vi "CreatePolynomial.vi"(6 "Save calibration":bool, 8 "Acquisition time (ms)":dbl=10000.0, 9 "Flyback (ms)":dbl=25.0, 10 "P(x)":dbl[](array[numeric])=[-0.257, 0.543, -0.0481, -0.0116] step=1e-10 format="%#.33f") -> (2 "Waveform Graph 2":dbl[](graph), 3 "Waveform Graph":dbl[](graph))   [LabVIEW 2020]
uses:
  <vilib>/Analysis/polynomials.llb/1D Polynomial Evaluation (DBL).vi
  <vilib>/Analysis/NI_AALPro.lvlib
panel:
  out "P(x) 2":dbl[](array[numeric])
  in  "Parameter string":string
  in  "Generate from string":bool
  out "size(s) 2":i32
  out "size(s)":i32
  out "x*y":dbl
  out "flyback min":dbl
  out "EndPosition":dbl
  out "InitialPosition":dbl
  # "=-0.257 + 0.543*F2 + -0.0481*F2^2 + -0.0116*F2^3"
  # "P(x) contains the real polynomial coefficients in ascending order of power."
  # "=-0.257 + 0.543*F2 + -0.0481*F2^2 + -0.0116*F2^3"
  # "D"
  # "C"
  # "B"
  # "A"
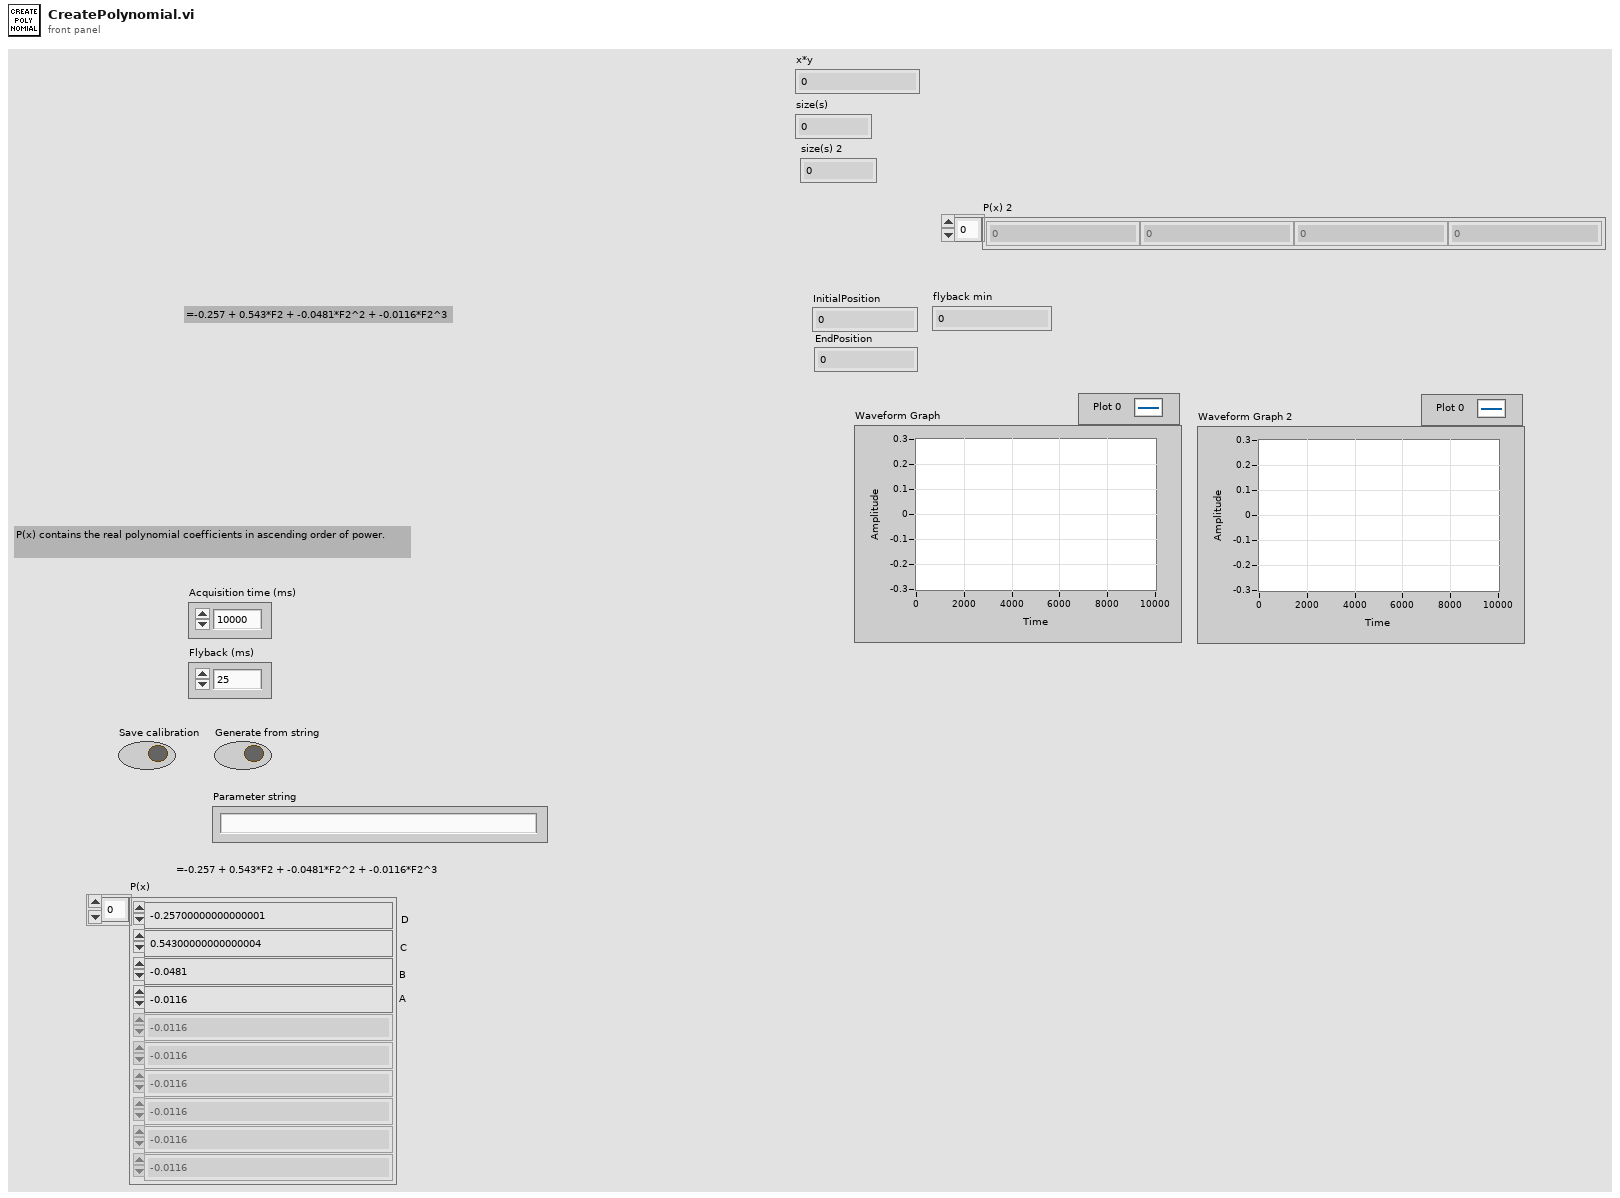
[diagram p1: front panel]
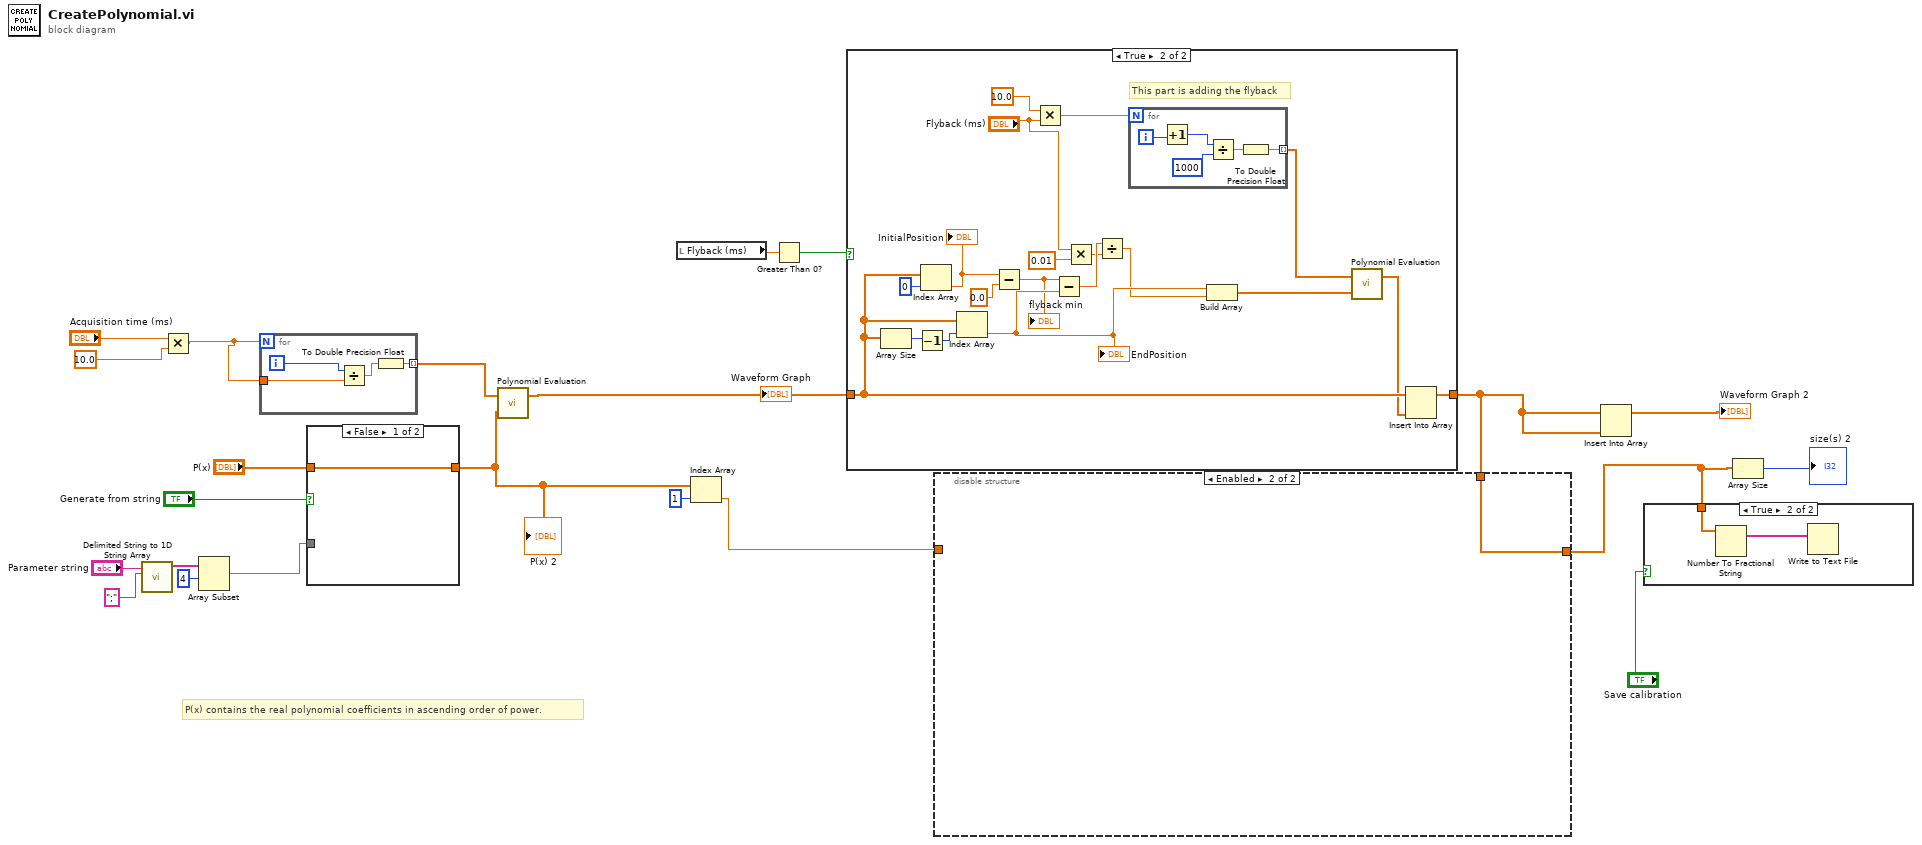
[diagram p0: block diagram]
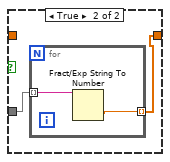
[diagram p3: hidden frame]
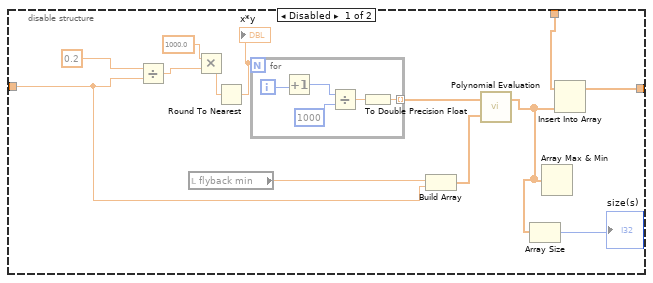
[diagram p4: hidden frame]
diagram:
  # "P(x) contains the real polynomial coefficients in ascending order of power."
  n1 = call <vilib>:"Delimited String to 1D String Array.vi"("delimiter"=";", "delimited string"="Parameter string") -> ("string array"=w6:string[])  [unwired: 9 in]
  n2 = Multiply(x="Acquisition time (ms)", y=10.0) -> (x*y=w18:dbl)
  n3 = Array Subset(array=w6, index=4) -> (w4:string[])  [unwired: 1 in]
  n4 = for {
    N: w18 -> [_]
    tunnel: [w26] -> w22 mode=indexing
    tunnel: w18 -> [w23]
    i -> [w25]
    n5 = Divide(x=w25, y=w23) -> (x/y=w24:dbl)
    n6 = To Double Precision Float(number=w24) -> (double precision float=w26:dbl)
  }
  n7 = case shown="False" "Generate from string" {
    tunnel: "P(x)" -> [w27 _]
    tunnel: [w27 w28] -> w9
    tunnel: w4 -> [_ w29]
    frame False {
    }
    frame True {
      n8 = for {
        tunnel: w29 -> [w31] mode=indexing
        tunnel: [w30] -> w28 mode=indexing
        n9 = Fract/Exp String To Number(string=w31) -> (number=w30:dbl)  [unwired: 3 in, 1 out]
      }
    }
  }
  "P(x) 2" <- w9
  n10 = call-poly <vilib>:"Polynomial Evaluation.vi"("P(x)"=w9, "A"=w22) -> ("P(A)"=w21:dbl[])  [unwired: 1 out]
  "Waveform Graph" <- w21
  n11 = local read "Flyback (ms)"() -> (w20:dbl)
  n12 = Index Array(array=w9, index=1) -> (element=w14:dbl)
  n13 = Greater Than 0?(x=w20) -> (x > 0?=w19:bool)
  n14 = case shown="True" w19 {
    tunnel: w21 -> [w32 w51]
    tunnel: [w32 w43] -> w2
    frame False {
    }
    frame True {
      # "This part is adding the flyback"
      n15 = Array Size(array=w51) -> (size(s)=w49:i32)
      n16 = Decrement(x=w49) -> (x-1=w48:i32)
      n17 = Index Array(array=w51, index=0) -> (element=w33:dbl)
      "InitialPosition" <- w33
      n18 = Index Array(array=w51, index=w48) -> (element=w41:dbl)
      "EndPosition" <- w41
      n19 = Subtract(x=w33, y=0.0) -> (x-y=w34:dbl)
      "flyback min" <- w34
      n20 = Multiply(x=10.0, y="Flyback (ms)") -> (x*y=w38:dbl)
      n21 = Subtract(x=w34, y=w41) -> (x-y=w42:dbl)
      n22 = Multiply(x="Flyback (ms)", y=0.01) -> (x*y=w39:dbl)
      n23 = Divide(x=w42, y=w39) -> (x/y=w40:dbl)
      n24 = for {
        N: w38 -> [_]
        tunnel: [w56] -> w45 mode=indexing
        i -> [w53]
        n25 = Increment(x=w53) -> (x+1=w52:i32)
        n26 = Divide(x=w52, y=1000) -> (x/y=w54:dbl)
        n27 = To Double Precision Float(number=w54) -> (double precision float=w56:dbl)
      }
      n28 = Build Array(w41, w40) -> (w47:dbl[])
      n29 = call-poly <vilib>:"Polynomial Evaluation.vi"("P(x)"=w47, "A"=w45) -> ("P(A)"=w44:dbl[])  [unwired: 1 out]
      n30 = Insert Into Array(array=w51, new element=w44) -> (w43:dbl[])  [unwired: 1 in]
    }
  }
  n31 = disable-structure shown="Enabled" {
    disable-tunnel: w2 -> [w69 w75]
    disable-tunnel: w14 -> [w58 _]
    disable-tunnel: [w57 w75] -> w12
    frame Disabled {
      n32 = Divide(x=0.2, y=w58) -> (x/y=w64:dbl)
      n33 = local read "flyback min"() -> (w65:dbl)
      n34 = Multiply(x=1000.0, y=w64) -> (x*y=w61:dbl)
      n35 = Round To Nearest(number=w61) -> (nearest integer value=w62:dbl)
      "x*y" <- w62
      n36 = for {
        N: w62 -> [_]
        tunnel: [w74] -> w67 mode=indexing
        i -> [w71]
        n37 = Increment(x=w71) -> (x+1=w70:i32)
        n38 = Divide(x=w70, y=1000) -> (x/y=w72:dbl)
        n39 = To Double Precision Float(number=w72) -> (double precision float=w74:dbl)
      }
      n40 = Build Array(w65, w58) -> (w66:dbl[])
      n41 = call-poly <vilib>:"Polynomial Evaluation.vi"("P(x)"=w66, "A"=w67) -> ("P(A)"=w60:dbl[])  [unwired: 1 out]
      n42 = Array Size(array=w60) -> (size(s)=→"size(s)":i32)
      n43 = Array Max & Min(array=w60) -> ()  [unwired: 4 out]
      n44 = Insert Into Array(array=w69, new element=w60) -> (w57:dbl[])  [unwired: 1 in]
    }
    frame Enabled {
    }
  }
  n45 = Insert Into Array(array=w2, new element=w2) -> (→"Waveform Graph 2":dbl[])  [unwired: 1 in]
  n46 = case shown="True" "Save calibration" {
    tunnel: w12 -> [_ w77]
    frame False {
    }
    frame True {
      n47 = Number To Fractional String(number=w77) -> (F-format string=w76:string[])  [unwired: 3 in]
      n48 = Write to Text File(text=w76) -> ()  [unwired: 3 in, 3 out]
    }
  }
  n49 = Array Size(array=w12) -> (size(s)=→"size(s) 2":i32)
